vi "485 comm GUID Lookup.vi"() -> ()   [LabVIEW 2016, in "485 comm Custom Device.lvlib"]
doc: "Use this Global VI to access the GUIDs assigned to the page resources of the Custom Device."
uses:
  485 comm Custom Device.lvlib
panel:
  in  "Custom Device":string="3931b391-e7b5-4179-b17a-553dbac04a5d"
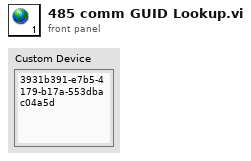
[diagram p1: front panel]
diagram:
